vi "Test_StreamToDisk_ValueOK.vi"(8 "error in (no error)":errorcluster, 11 "TestCase in":refnum<class "TestTransport.lvclass">) -> (0 "error out":errorcluster, 3 "TestCase out":refnum<class "TestTransport.lvclass">)   [LabVIEW 2017, in "TestTransport.lvclass"]
uses:
  TestTransport.lvclass
  <vilib>/Utility/sysdir.llb/System Directory Type.ctl
  StreamToDiskTransport/StreamToDiskTransport.lvclass/StreamToDiskTransport.ctl
  <vilib>/Utility/error.llb/Clear Errors.vi
  StreamToDiskTransport/StreamToDiskTransport.lvclass
panel:
  out "Test File Path":path
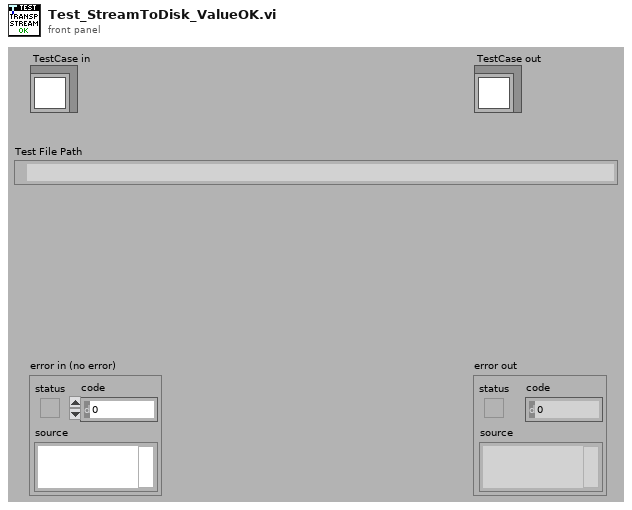
[diagram p1: front panel]
types:
  T1 = enum16{"open", "open or create", "create or replace", "create", "open (read-only)"}
  T2 = typedef "System Directory Type.ctl" = i32
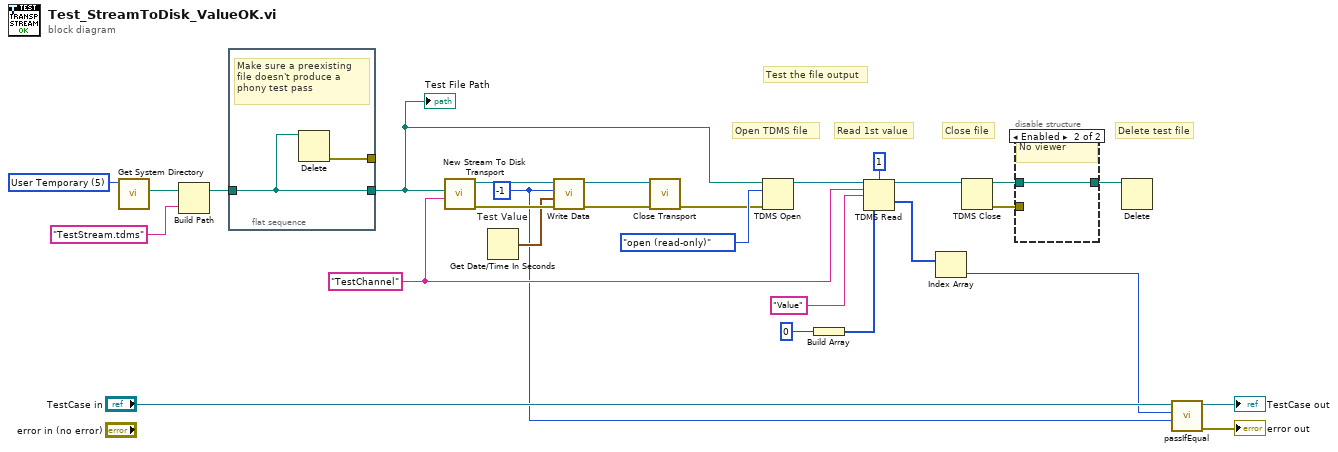
[diagram p0: block diagram]
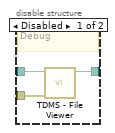
[diagram p2: hidden frame]
diagram:
  w1 = -1  # Test Value
  w17 = "TestChannel" ("Channel Name")
  w23 = T2 5 items=["User Home"=0, "User Desktop"=1, "User Documents"=2, "User Application Data"=3, "User Preferences"=4, "User Temporary"=5, "Public Documents"=6, "Public Application Data"=7, "Public Preferences"=8, "Public Cache"=13, "System Core Libraries"=9, "System Installed Libraries"=10, "Application Files"=11, "Boot Volume Root"=12] ("system directory type")
  # "Close file"
  # "Open TDMS file"
  # "Delete test file"
  # "Test the file output"
  # "Read 1st value"
  n1 = call <vilib>:"Get System Directory.vi"("system directory type"=w23) -> ("system directory"=w22:path)  [unwired: 10 in]
  n2 = Build Path(base path=w22, name or relative path="TestStream.tdms") -> (appended path=w3:path)
  n3 = flat-sequence {
    tunnel: w3 -> [w30]
    tunnel: [w30] -> w2
    tunnel: [w29] -> _
    frame #0 {
      # "Make sure a preexisting\nfile doesn't produce a\nphony test pass"
      n4 = Delete(path (use dialog)=w30) -> (error out=w29:errorcluster)  [unwired: 4 in, 2 out]
    }
  }
  n5 = call "New Stream To Disk Transport.vi"("Channel Name"=w17, "File Path"=w2) -> ("error out"=w24:errorcluster, "StreamToDiskTransport"=w25:refnum<class "StreamToDiskTransport.lvclass">)  [unwired: 8 in]
  n6 = Get Date/Time In Seconds() -> (seconds since 1Jan1904=w16:timestamp)
  n7 = call-dynamic "Write Data.vi"("error in (no error)"=w24, "Publication Time"=w16, "Value"=w1, "StreamToDiskTransport In"=w25) -> ("error out"=w19:errorcluster, "StreamToDiskTransport Out"=w20:refnum<class "StreamToDiskTransport.lvclass">)  [unwired: 6 in]
  n8 = call-dynamic "Close Transport.vi"("error in (no error)"=w19, "StreamToDiskTransport"=w20) -> ("error out"=w4:errorcluster)  [unwired: 9 in]
  n9 = TDMS Open(8:w4, 10:T1."open (read-only)" ("operation (0:open)"), 11:w2) -> (3:w15:refnum<k34>)  [unwired: 4 in, 1 out]
  n10 = Build Array(0) -> (w11:i32[])
  n11 = TDMS Read(0:w15, 2:i64 1 ("count (-1: all)"), 5:w17, 7:"Value" ("channel name(s) in"), 12:w11) -> (4:w10:refnum<k34>, 10:w8:i32[])  [unwired: 3 in, 4 out]
  n12 = Index Array(array=w8) -> (element=w7:i32)  [unwired: 1 in]
  n13 = TDMS Close(11:w10) -> (0:w6:errorcluster, 3:w9:path)  [unwired: 1 in]
  n14 = disable-structure shown="Enabled" {
    disable-tunnel: [w33 w34] -> w18
    disable-tunnel: w9 -> [w32 w34]
    disable-tunnel: w6 -> [w31 _]
    frame Disabled {
      # "Debug"
      n15 = call <vilib>:"TDMS - File Viewer.vi"("error in (no error)"=w31, "file path"=w32) -> ("file path out"=w33:path)  [unwired: 4 in, 1 out]
    }
    frame Enabled {
      # "No viewer"
    }
  }
  n16 = Delete(path (use dialog)=w18) -> ()  [unwired: 4 in, 3 out]
  n17 = call-dynamic "passIfEqual.vi"("y"=w1, "x"=w7, "TestCase in"="TestCase in") -> ("error out"=→"error out":errorcluster, "TestCase out"=→"TestCase out":refnum<class "TestTransport.lvclass">)  [unwired: 7 in]
  "Test File Path" <- w2
